vi "Parce DO CMD.vi"(0 "CMD":u64) -> (4 "#DO":u8, 6 "Value":bool, 8 "Time uSec":u32)   [LabVIEW 2019]
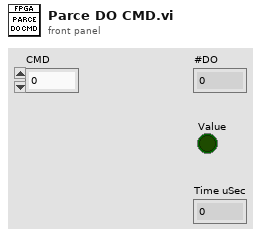
[diagram p1: front panel]
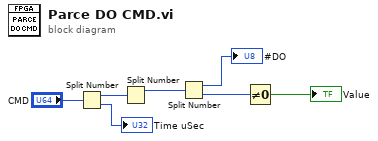
[diagram p0: block diagram]
diagram:
  n1 = Split Number(x="CMD") -> (hi(x)=w6:u32, lo(x)=→"Time uSec":u32)
  n2 = Split Number(x=w6) -> (hi(x)=w5:u16)  [unwired: 1 out]
  n3 = Split Number(x=w5) -> (hi(x)=→"#DO":u8, lo(x)=w3:u8)
  n4 = Not Equal To 0?(x=w3) -> (x != 0?=→"Value":bool)
